vi "to string 1.0.vi"(8 "error in (no error)":errorcluster, 10 "data in":string, 11 "Multiplexer configuration in":refnum<class "Multiplexer configuration.lvclass">) -> (0 "error out":errorcluster, 2 "data out":string, 3 "Multiplexer configuration out":refnum<class "Multiplexer configuration.lvclass">)   [LabVIEW 2021, in "Multiplexer configuration.lvclass"]
uses:
  Multiplexer configuration.lvclass
  Multiplexer configuration.lvclass/Multiplexer configuration.ctl
  <vilib>/NI/Tag Bus Module Framework/channel/TBM channel.lvclass
  <vilib>/NI/Configuration Framework/serializable configuration/NISE_CEF_serializable configuration.lvclass
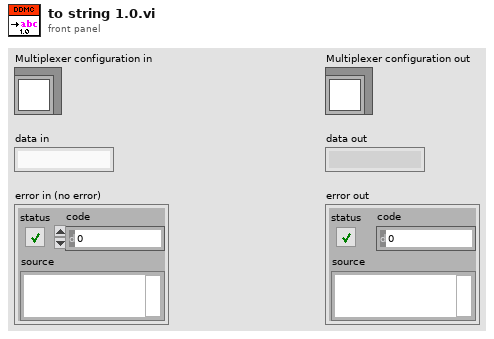
[diagram p1: front panel]
types:
  T1 = typedef "Multiplexer configuration.lvclass/Line.ctl" = cluster{"A":refnum<class "TBM channel.lvclass">, "B":refnum<class "TBM channel.lvclass">, "Select":refnum<class "TBM channel.lvclass">, "Output":refnum<class "TBM channel.lvclass">}
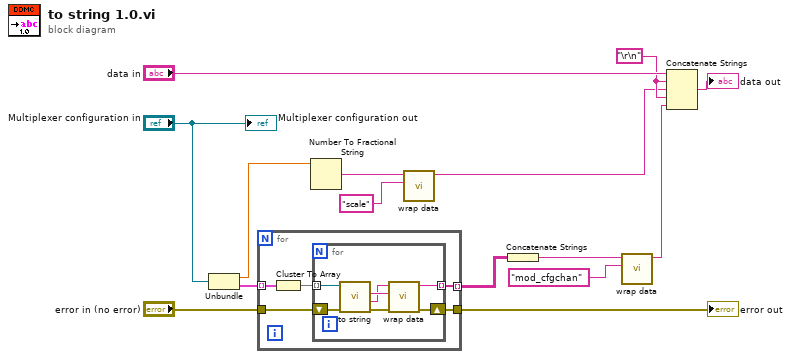
[diagram p0: block diagram]
diagram:
  w2 = "\r\n"
  n1 = Unbundle("Multiplexer configuration in") -> (w3:dbl, w4:T1[])
  n2 = for {
    tunnel: w4 -> [w20] mode=indexing
    tunnel: [w18] -> w8 mode=indexing
    tunnel: "error in (no error)" -> [w17]
    tunnel: [w16] -> w15
    n3 = Cluster To Array(cluster=w20) -> (array=w19:refnum<class "TBM channel.lvclass">[])
    n4 = for {
      tunnel: w19 -> [w26] mode=indexing
      tunnel: [w23] -> w18 mode=indexing
      shift-right: [w21] -> w16
      shift-left: w17 -> [w22]
      n5 = call-dynamic "to string.vi"("error in"=w22, "channel in"=w26) -> ("error out"=w21:errorcluster, "channel data"=w24:string, "identifier"=w25:string)  [unwired: 6 in, 1 out]
      n6 = call <vilib>:"wrap data.vi"("identifier"=w25, "data to wrap"=w24) -> ("wrapped data"=w23:string)  [unwired: 9 in]
    }
  }
  "error out" <- w15
  n7 = Number To Fractional String(number=w3) -> (F-format string=w5:string)  [unwired: 3 in]
  n8 = call <vilib>:"wrap data.vi"("identifier"="scale", "data to wrap"=w5) -> ("wrapped data"=w1:string)  [unwired: 9 in]
  n9 = Concatenate Strings(w8) -> (w9:string)
  n10 = call <vilib>:"wrap data.vi"("identifier"="mod_cfgchan", "data to wrap"=w9) -> ("wrapped data"=w12:string)  [unwired: 9 in]
  n11 = Concatenate Strings("data in", w2, w1, w2, w12) -> (→"data out":string)
  "Multiplexer configuration out" <- "Multiplexer configuration in"
